vi "Select FPGA.vi"(8 "error in":errorcluster, 11 "Item Ref in":T12 format="%.0x") -> (0 "error out":errorcluster, 1 "FPGA Info":T10, 2 "FPGA Reference":T12=18446744073709551615 format="%.0x", 3 "Item Ref out":T12 format="%.0x", 4 "Cancelled?":bool, 5 "VS FPGA?":bool, 7 "Bitfile Path out":path)   [LabVIEW 2011, in "Engine Sim System Explorer.lvlib"]
uses:
  Engine Sim System Explorer.lvlib
  <vilib>/NI Veristand/Custom Device API/Custom Device Item Ref.ctl
  TypeDefs/EngineSimComps.ctl
  TypeDefs/APUComp.ctl
  TypeDefs/NTeethComp.ctl
  TypeDefs/FullyCustomComp.ctl
  Shared/FullyCustomCommMode.ctl
  TypeDefs/FullyCustomProfilesComp.ctl
  TypeDefs/ECUEventComp.ctl
  TypeDefs/DataReplayLoopComp.ctl
  TypeDefs/DataReplayComp.ctl
  <userlib>/_FPGA Interface Advanced Tools/FPGA Bitfile Utility/TypeDefs/Scalar Register Set.ctl
  <userlib>/_FPGA Interface Advanced Tools/FPGA Bitfile Utility/TypeDefs/Scalar Register.ctl
  <userlib>/_FPGA Interface Advanced Tools/FPGA Bitfile Utility/TypeDefs/Array Register Set.ctl
  <userlib>/_FPGA Interface Advanced Tools/FPGA Bitfile Utility/TypeDefs/Array Register.ctl
  <userlib>/_FPGA Interface Advanced Tools/FPGA Bitfile Utility/TypeDefs/FIFO Channel Set.ctl
  <userlib>/_FPGA Interface Advanced Tools/FPGA Bitfile Utility/TypeDefs/FIFO Channel.ctl
  <vilib>/NI Veristand/Custom Device Tools/Custom Device Utility Library/Custom Device Utility Library.lvlib
  <vilib>/NI Veristand/Custom Device API/Custom Device API.lvlib
  <userlib>/_FPGA Interface Advanced Tools/FPGA Bitfile Utility/FPGA Bitfile Utility.lvlib
  Engine Simulation Shared.lvlib
panel:
  in  "Bitfile Path":path
  in  "Cancel":bool
  in  "FPGA Selection Type":T11(radio)
  in  "OK":bool
  in  "RIO Device Address":u16(ring)
  in  "RIO Device Address":string="RIO0"
  # "Invalid Bitfile!"
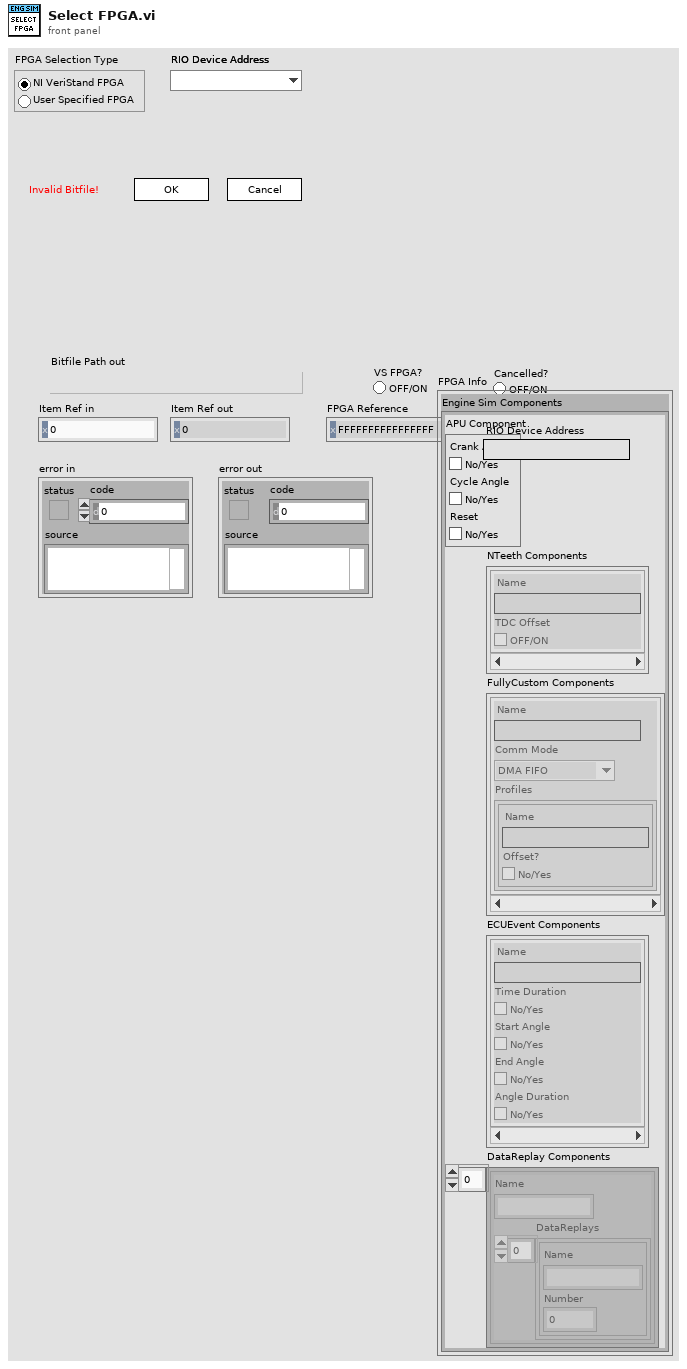
[diagram p1: front panel]
types:
  T1 = typedef "Engine Sim System Explorer.lvlib/EngineSimComps.ctl" = cluster{"APU Component":T2, "NTeeth Components":T3[], "FullyCustom Components":T4[], "ECUEvent Components":T7[], "DataReplay Components":T8[]}
  T2 = typedef "Engine Sim System Explorer.lvlib/APUComp.ctl" = cluster{"Crank Angle":bool, "Cycle Angle":bool, "Reset":bool}
  T3 = typedef "Engine Sim System Explorer.lvlib/NTeethComp.ctl" = cluster{"Name":string, "TDC Offset":bool}
  T4 = typedef "Engine Sim System Explorer.lvlib/FullyCustomComp.ctl" = cluster{"Name":string, "Comm Mode":T5, "Profiles":T6[]}
  T5 = typedef "Engine Simulation Shared.lvlib/FullyCustomCommMode.ctl" = enum16{"DMA FIFO", "FP Data Transfer"}
  T6 = typedef "Engine Sim System Explorer.lvlib/FullyCustomProfilesComp.ctl" = cluster{"Name":string, "Offset?":bool}
  T7 = typedef "Engine Sim System Explorer.lvlib/ECUEventComp.ctl" = cluster{"Name":string, "Time Duration":bool, "Start Angle":bool, "End Angle":bool, "Angle Duration":bool}
  T8 = typedef "Engine Sim System Explorer.lvlib/DataReplayLoopComp.ctl" = cluster{"Name":string, "DataReplays":T9[]}
  T9 = typedef "Engine Sim System Explorer.lvlib/DataReplayComp.ctl" = cluster{"Name":string, "Number":u8}
  T10 = cluster{"RIO Device Address":string, "Engine Sim Components":T1}
  T11 = enum32{"NI VeriStand FPGA", "User Specified FPGA"}
  T12 = typedef "Custom Device API.lvlib/Custom Device Item Ref.ctl" = u64
  T13 = enum8{"Enabled", "Disabled", "Disabled and Grayed Out"}
  T14 = typedef "FPGA Bitfile Utility.lvlib/Scalar Register Set.ctl" = cluster{"Boolean":T15[], "I8":T15[], "I16":T15[], "I32":T15[], "I64":T15[], "U8":T15[], "U16":T15[], "U32":T15[], "U64":T15[]}
  T15 = typedef "FPGA Bitfile Utility.lvlib/Scalar Register.ctl" = cluster{"Address":u32, "Name":string}
  T16 = typedef "FPGA Bitfile Utility.lvlib/Array Register Set.ctl" = cluster{"Boolean":T17[], "I8":T17[], "I16":T17[], "I32":T17[], "I64":T17[], "U8":T17[], "U16":T17[], "U32":T17[], "U64":T17[]}
  T17 = typedef "FPGA Bitfile Utility.lvlib/Array Register.ctl" = cluster{"Address":u32, "Num Elements":u32, "Name":string}
  T18 = typedef "FPGA Bitfile Utility.lvlib/FIFO Channel Set.ctl" = cluster{"Boolean":T19[], "I8":T19[], "I16":T19[], "I32":T19[], "I64":T19[], "U8":T19[], "U16":T19[], "U32":T19[], "U64":T19[]}
  T19 = typedef "FPGA Bitfile Utility.lvlib/FIFO Channel.ctl" = cluster{"Physical Channel":u32, "Name":string}
  T20 = cluster{"Indicator Scalars":T14, "Control Scalars":T14, "Control Arrays":T16, "HostToTarget":T18}[]
  T21 = cluster{"Indicator Scalars":T14, "Control Scalars":T14, "Control Arrays":T16, "HostToTarget":T18}
  T22 = typedef "Custom Device API.lvlib/Custom Device Item Info.ctl" = cluster{"Name":string, "Is Channel":bool, "GUID":string}
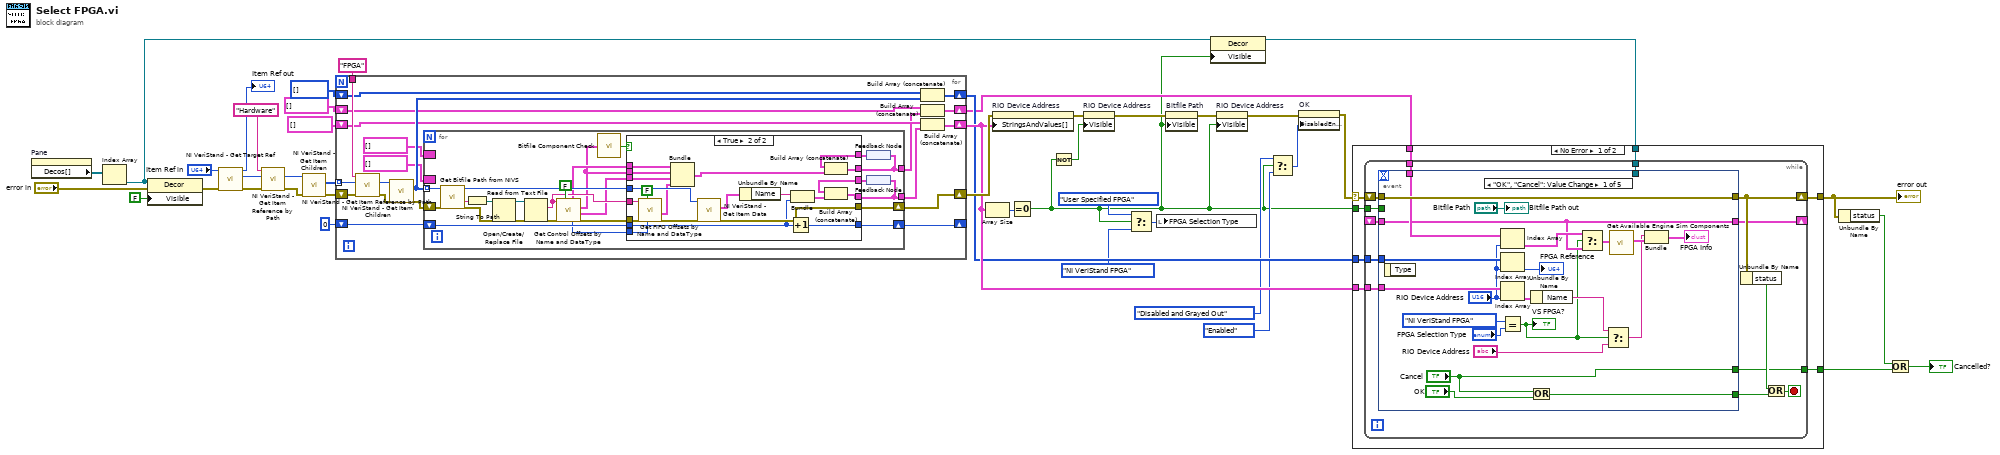
[diagram p0: block diagram]
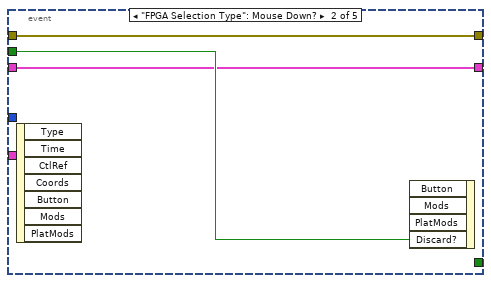
[diagram p2: hidden frame]
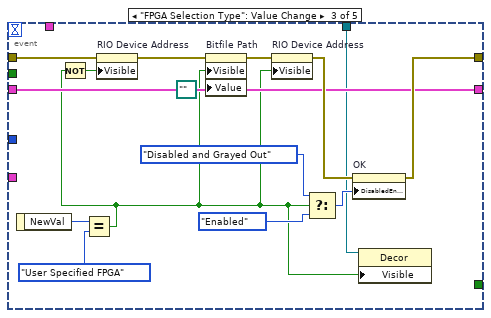
[diagram p3: hidden frame]
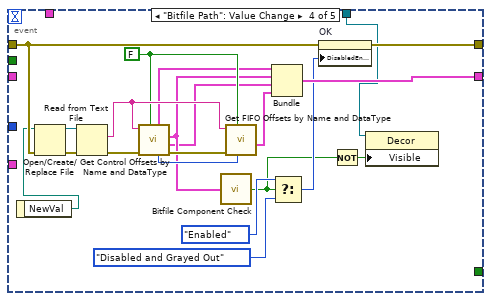
[diagram p4: hidden frame]
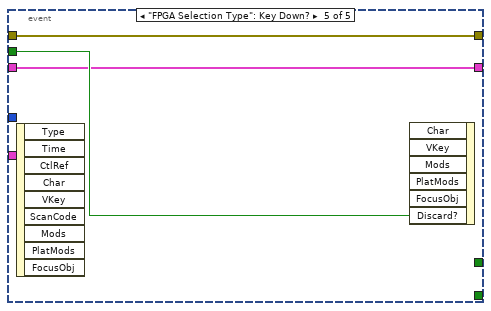
[diagram p5: hidden frame]
diagram:
  n1 = property on="Pane" class="Pane"() -> ("Decos[]"=w8:refnum<vi>[])  [unwired: 2 in, 2 out]
  n2 = Index Array(array=w8) -> (element=w4:refnum<vi>)  [unwired: 1 in]
  n3 = property class="Decor"(reference=w4, error in="error in", "Visible"=FALSE) -> (error out=w5:errorcluster)  [unwired: 1 out]
  n4 = call <vilib>:"NI VeriStand - Get Target Ref.vi"("error in"=w5, "Item Ref in"="Item Ref in") -> ("error out"=w38:errorcluster, "Target Ref"=w42:T12, "Item Ref out"=→"Item Ref out":T12)  [unwired: 6 in, 1 out]
  n5 = call <vilib>:"NI VeriStand - Get Item Reference by Path.vi"("error in (no error)"=w38, "Root Ref"=w42, "Item Path in"="Hardware") -> ("error out"=w39:errorcluster, "Item Ref"=w40:T12)  [unwired: 5 in, 2 out]
  n6 = call <vilib>:"NI VeriStand - Get Item Children.vi"("error in (no error)"=w39, "Item Ref in"=w40) -> ("error out"=w35:errorcluster, "Child Refs"=w37:T12[])  [unwired: 6 in, 2 out]
  n7 = for {
    tunnel: w37 -> [w62] mode=indexing
    tunnel: "FPGA" ("Item Path in") -> [w61]
    shift-right: [w50] -> w34
    shift-left: w35 -> [w59]
    shift-right: [w54] -> w26
    shift-left: T12[] [] -> [w53]
    shift-right: [w52] -> w27
    shift-left: cluster{"Name":string, u16}[] [] -> [w51]
    shift-right: [w49] -> _
    shift-left: u16 0 -> [w48]
    shift-right: [w46] -> w13
    shift-left: T20 [] -> [w45]
    n8 = call <vilib>:"NI VeriStand - Get Item Reference by Path.vi"("error in (no error)"=w59, "Root Ref"=w62, "Item Path in"=w61) -> ("error out"=w58:errorcluster, "Item Ref"=w60:T12)  [unwired: 5 in, 2 out]
    n9 = call <vilib>:"NI VeriStand - Get Item Children.vi"("error in (no error)"=w58, "Item Ref in"=w60) -> ("error out"=w57:errorcluster, "Child Refs"=w55:T12[])  [unwired: 6 in, 2 out]
    n10 = for {
      tunnel: w55 -> [w83] mode=indexing
      tunnel: [w67] -> w56
      shift-right: [w86] -> w50
      shift-left: w57 -> [w82]
      shift-right: [w85] -> w49
      shift-left: w48 -> [w84]
      border: cluster{"Name":string, u16}[] [] -> [_]
      border: T20 [] -> [_]
      tunnel: [w65] -> w44
      n11 = call "Get Bitfile Path from NIVS.vi"("error in (no error)"=w82, "ID in"=w83) -> ("error out"=w78:errorcluster, "Path"=w80:string, "ID out"=w81:T12)  [unwired: 7 in]
      n12 = String To Path(string=w80) -> (path=w79:path)
      n13 = Open/Create/Replace File(file path (use dialog)=w79, error in=w78) -> (refnum out=w76:refnum<file>, error out=w77:errorcluster)  [unwired: 4 in, 1 out]
      n14 = Read from Text File(file (use dialog)=w76, error in=w77) -> (text=w73:string, error out=w75:errorcluster)  [unwired: 2 in, 2 out]
      n15 = call <userlib>:"Get Control Offsets by Name and DataType.vi"("User Specified?"=FALSE, "error in"=w75, "bitfile xml in"=w73) -> ("error out"=w72:errorcluster, "Control Arrays"=w63:T16, "Control Scalars"=w68:T14, "offset past EndTag"=w71:i32, "Indicator Scalars"=w69:T14)  [unwired: 3 in, 1 out]
      n16 = call "Bitfile Component Check.vi"("Control Scalars"=w68) -> ("Valid?"=w70:bool)
      n17 = feedback #1() -> (w64:T20)
      n18 = feedback #2() -> (w66:cluster{"Name":string, u16}[])
      n19 = case shown="True" w70 {
        tunnel: [w89 w109] -> w86
        tunnel: [w90 w99] -> w67
        tunnel: [w88 w107] -> w85
        tunnel: w84 -> [w88 w106]
        tunnel: w81 -> [_ w105]
        tunnel: w73 -> [_ w104]
        tunnel: w72 -> [w89 w103]
        tunnel: w71 -> [_ w102]
        tunnel: w69 -> [_ w98]
        tunnel: w68 -> [_ w97]
        tunnel: [w87 w95] -> w65
        tunnel: w66 -> [w90 w94]
        tunnel: w64 -> [w87 w93]
        tunnel: w63 -> [_ w92]
        frame False {
        }
        frame True {
          n20 = call <userlib>:"Get FIFO Offsets by Name and DataType.vi"("offset"=w102, "User Specified?"=FALSE, "error in"=w103, "bitfile xml in"=w104) -> ("error out"=w100:errorcluster, "HostToTarget"=w96:T18)  [unwired: 3 in, 3 out]
          n21 = Bundle("Indicator Scalars"=w98, "Control Scalars"=w97, "Control Arrays"=w92, "HostToTarget"=w96) -> (w91:T21)  [unwired: 1 in]
          n22 = call <vilib>:"NI VeriStand - Get Item Data.vi"("error in (no error)"=w100, "Item Ref in"=w105) -> ("error out"=w109:errorcluster, "Item Info"=w111:T22)  [unwired: 6 in, 2 out]
          n23 = Unbundle By Name(w111) -> ("Name"=w110:string)
          n24 = Increment(x=w106) -> (x+1=w107:u16)
          n25 = Bundle("Name"=w110, w106) -> (w108:cluster{"Name":string, u16})  [unwired: 1 in]
          n26 = Build Array (concatenate)(w93, w91) -> (w95:T20)
          n27 = Build Array (concatenate)(w94, w108) -> (w99:cluster{"Name":string, u16}[])
        }
      }
      n28 = feedback-in #1(w65) -> ()
      n29 = feedback-in #2(w67) -> ()
    }
    n30 = Build Array (concatenate)(w53, w55) -> (w54:T12[])
    n31 = Build Array (concatenate)(w45, w44) -> (w46:T20)
    n32 = Build Array (concatenate)(w51, w56) -> (w52:cluster{"Name":string, u16}[])
  }
  n33 = Array Size(array=w27) -> (size(s)=w28:i32)
  n34 = property on="RIO Device Address" class="Ring (strict)"(error in=w34, "StringsAndValues[]"=w27) -> (error out=w25:errorcluster)  [unwired: 1 in, 1 out]
  n35 = Equal To 0?(x=w28) -> (x = 0?=w3:bool)
  n36 = Not(x=w3) -> (.not. x?=w24:bool)
  n37 = property on="RIO Device Address" class="Ring (strict)"(error in=w25, "Visible"=w24) -> (error out=w23:errorcluster)  [unwired: 1 in, 1 out]
  n38 = Select(t=T11."User Specified FPGA" ("x"), s=w3, f=T11."NI VeriStand FPGA" ("x")) -> (s? t:f=w21:T11)
  n39 = local write "FPGA Selection Type"(w21) -> ()
  n40 = property on="Bitfile Path" class="Path"(error in=w23, "Visible"=w3) -> (error out=w22:errorcluster)  [unwired: 1 in, 1 out]
  n41 = property class="Decor"(reference=w4, "Visible"=w3) -> (reference out=w2:refnum<vi>)  [unwired: 1 in, 1 out]
  n42 = property on="RIO Device Address" class="Str"(error in=w22, "Visible"=w3) -> (error out=w17:errorcluster)  [unwired: 1 in, 1 out]
  n43 = Select(t=T13."Disabled and Grayed Out" ("Disabled"), s=w3, f=T13."Enabled" ("Disabled")) -> (s? t:f=w14:T13)
  n44 = property on="OK" class="Bool"(error in=w17, "DisabledEnum"=w14) -> (error out=w1:errorcluster)  [unwired: 1 in, 1 out]
  n45 = case shown="No Error" w1 {
    selector: w1 -> [w116 w197]
    tunnel: w27 -> [w119 _]
    tunnel: w26 -> [w118 _]
    tunnel: w3 -> [w117 _]
    tunnel: [w115 w197] -> w10
    tunnel: w13 -> [w114 _]
    tunnel: [w113 _] -> w11
    tunnel: w2 -> [w112 _]
    frame No Error {
      n46 = while {
        tunnel: w117 -> [w129]
        tunnel: w119 -> [w131]
        tunnel: w118 -> [w130]
        shift-right: [w126] -> w115
        shift-left: w116 -> [w128]
        shift-right: [w125] -> _
        shift-left: _ -> [w124]
        tunnel: w114 -> [w123]
        tunnel: [w121] -> w113
        tunnel: w112 -> [w120]
        stop <- w127 stop-if-true
        n47 = event shown="[0] \"OK\", \"Cancel\": Value Change" {
          selector: _ -> [_ _ _ _ _]
          dyn-events: _ -> [_ _ _ _ _]
          timeout: _ -> [_ _ _ _ _]
          tunnel: [w153 _ _ _ _] -> w132
          tunnel: w131 -> [w151 _ _ _ _]
          tunnel: w130 -> [w145 _ _ _ _]
          tunnel: w129 -> [_ w157 _ _ w196]
          tunnel: w128 -> [w143 w156 w170 w183 w195]
          tunnel: [w143 w156 w166 w184 w195] -> w126
          tunnel: [w139 w155 w164 w182 w194] -> w125
          tunnel: w124 -> [w139 w155 w164 _ w194]
          tunnel: w123 -> [w141 _ _ _ _]
          tunnel: ["Cancel" _ _ _ _] -> w121
          tunnel: w120 -> [_ _ w159 w175 _]
          event "OK", "Cancel": Value Change {
            n48 = event-data() -> ()  [unwired: 1 in, 1 out]
            n49 = Index Array(array=w141, index="RIO Device Address") -> (element=w140:T21)
            n50 = Index Array(array=w145, index="RIO Device Address") -> (element=→"FPGA Reference":T12)
            n51 = Index Array(array=w151, index="RIO Device Address") -> (element=w150:cluster{"Name":string, u16})
            n52 = Equal?(x=T11."NI VeriStand FPGA", y="FPGA Selection Type") -> (x = y?=w138:bool)
            "VS FPGA?" <- w138
            n53 = Or(x="Cancel", y="OK") -> (x .or. y?=w153:bool)
            n54 = Unbundle By Name(w150) -> ("Name"=w149:string)
            n55 = Select(t=w140, s=w138, f=w139) -> (s? t:f=w137:T21)
            n56 = Select(t=w149, s=w138, f="RIO Device Address") -> (s? t:f=w134:string)
            n57 = call "Get Available Engine Sim Components.vi"("Register info"=w137) -> ("Engine Sim Components"=w135:T1)  [unwired: 10 in]
            n58 = Bundle("RIO Device Address"=w134, "Engine Sim Components"=w135) -> (→"FPGA Info":T10)  [unwired: 1 in]
            "Bitfile Path out" <- "Bitfile Path"
          }
          event "FPGA Selection Type": Mouse Down? {
            n59 = event-data() -> ()  [unwired: 1 in, 7 out]
            n60 = event-data("Discard?"=w157) -> ()  [unwired: 4 in, 1 out]
          }
          event "FPGA Selection Type": Value Change {
            n61 = event-data() -> ("NewVal"=w169:T11)  [unwired: 1 in]
            n62 = Equal?(x=w169, y=T11."User Specified FPGA" ("x")) -> (x = y?=w160:bool)
            n63 = Not(x=w160) -> (.not. x?=w167:bool)
            n64 = property on="RIO Device Address" class="Ring (strict)"(error in=w170, "Visible"=w167) -> (error out=w171:errorcluster)  [unwired: 1 in, 1 out]
            n65 = property on="Bitfile Path" class="Path"(error in=w171, "Visible"=w160, "Value"=path "" ("Bitfile Path")) -> (error out=w172:errorcluster)  [unwired: 1 in, 1 out]
            n66 = property on="RIO Device Address" class="Str"(error in=w172, "Visible"=w160) -> (error out=w165:errorcluster)  [unwired: 1 in, 1 out]
            n67 = Select(t=T13."Disabled and Grayed Out" ("Disabled"), s=w160, f=T13."Enabled" ("Disabled")) -> (s? t:f=w161:T13)
            n68 = property on="OK" class="Bool"(error in=w165, "DisabledEnum"=w161) -> (error out=w166:errorcluster)  [unwired: 1 in, 1 out]
            n69 = property class="Decor"(reference=w159, "Visible"=w160) -> ()  [unwired: 1 in, 2 out]
          }
          event "Bitfile Path": Value Change {
            w191 = FALSE ("User Specified?")
            n70 = event-data() -> ("NewVal"=w178:path)  [unwired: 1 in]
            n71 = Open/Create/Replace File(file path (use dialog)=w178, error in=w183) -> (refnum out=w188:refnum<file>, error out=w189:errorcluster)  [unwired: 4 in, 1 out]
            n72 = Read from Text File(file (use dialog)=w188, error in=w189) -> (text=w193:string, error out=w174:errorcluster)  [unwired: 2 in, 2 out]
            n73 = call <userlib>:"Get Control Offsets by Name and DataType.vi"("User Specified?"=w191, "error in"=w174, "bitfile xml in"=w193) -> ("error out"=w190:errorcluster, "Control Arrays"=w173:T16, "Control Scalars"=w186:T14, "offset past EndTag"=w192:i32, "Indicator Scalars"=w185:T14)  [unwired: 3 in, 1 out]
            n74 = call "Bitfile Component Check.vi"("Control Scalars"=w186) -> ("Valid?"=w176:bool)
            n75 = call <userlib>:"Get FIFO Offsets by Name and DataType.vi"("offset"=w192, "User Specified?"=w191, "error in"=w190, "bitfile xml in"=w193) -> ("HostToTarget"=w187:T18)  [unwired: 3 in, 4 out]
            n76 = Bundle("Indicator Scalars"=w185, "Control Scalars"=w186, "Control Arrays"=w173, "HostToTarget"=w187) -> (w182:T21)  [unwired: 1 in]
            n77 = Select(t=T13."Enabled" ("Disabled"), s=w176, f=T13."Disabled and Grayed Out" ("Disabled")) -> (s? t:f=w179:T13)
            n78 = property on="OK" class="Bool"(error in=w183, "DisabledEnum"=w179) -> (error out=w184:errorcluster)  [unwired: 1 in, 1 out]
            n79 = Not(x=w176) -> (.not. x?=w177:bool)
            n80 = property class="Decor"(reference=w175, "Visible"=w177) -> ()  [unwired: 1 in, 2 out]
          }
          event "FPGA Selection Type": Key Down? {
            n81 = event-data() -> ()  [unwired: 1 in, 9 out]
            n82 = event-data("Discard?"=w196) -> ()  [unwired: 6 in, 1 out]
          }
        }
        n83 = Unbundle By Name(w126) -> ("status"=w122:bool)
        n84 = Or(x=w122, y=w132) -> (x .or. y?=w127:bool)
      }
    }
    frame Error {
    }
  }
  "error out" <- w10
  n85 = Unbundle By Name(w10) -> ("status"=w9:bool)
  n86 = Or(x=w9, y=w11) -> (x .or. y?=→"Cancelled?":bool)
